vi "User Interface.vi"(10 "Test File Path":path=path "") -> ()   [LabVIEW 2020, in "Execution UI.lvclass"]
uses:
  Execution UI.lvclass
  Execution UI.lvclass/Execution UI.ctl
  <vilib>/Utility/miscctls.llb/LVNodeAndColumnTypeDef.ctl
  Private/TypeDefs/Execution State.ctl
  <vilib>/Platform/browser.llb/Open URL in Default Browser (string).vi
  Core/Result/Status.ctl
  Core/Result/Result.lvlib
  Result Model/Result Model.lvclass
  Core/Result/Type.ctl
  Core/Result/Result.ctl
  Framework/Test Finder/Test Finder.lvclass
  Framework/Test Runner/Test Runner.lvclass
  Configuration Manager/UI Configuration Manager.lvclass
  Result Model/Tree Item Filter.ctl
  Private/TypeDefs/Virtual Key.ctl
  Framework/Plugin/Plugin.lvclass
panel:
  in  "Refresh":bool
  in  "Run Selected Tests":bool
  in  "Stop":bool
  in  "Run All Tests":bool
  in  "Eject":bool
  in  "Collapse":bool
  in  "Expand":bool
  out "Progress bar":dbl(slide) scale=0.0..100.0
  out "Results":i32(listbox)=-1
  in  "Test Results":string[](tree)
  out "Shift?":bool
  in  "Filter fails":bool
  out "Description":string
  out "Status":string
  # "1"
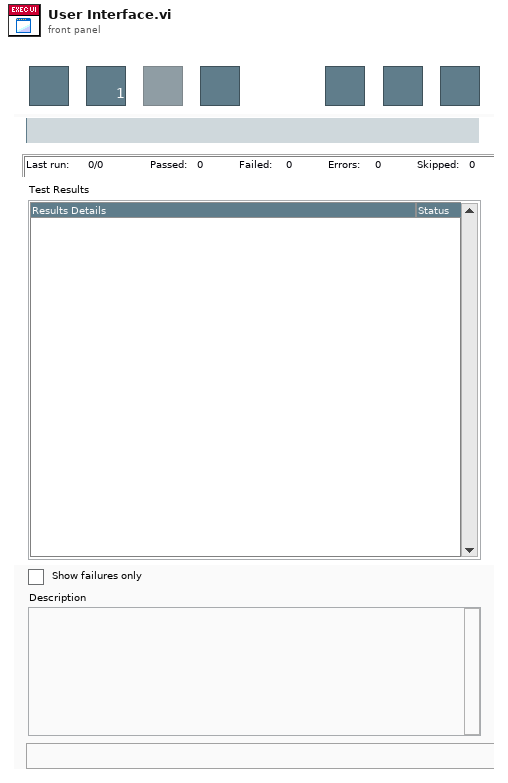
[diagram p1: front panel]
types:
  T1 = typedef "LVNodeAndColumnTypeDef.ctl" = cluster{"Node":string, "Column":i32}
  T2 = typedef "Result Model.lvclass/Tree Item Filter.ctl" = enum16{"All", "Only Fails", "Fails or else Not Executed"}
  T3 = cluster{"Text.Selection":cluster{"Selection Start":u32, "Selection End":u32}, "Color":u32}
  T4 = enum32{"Invalid", "Standard", "Closed", "Hidden", "Minimized", "Maximized"}
  T5 = typedef "Execution UI.lvclass/Execution State.ctl" = enum16{"Idle", "Running"}
  T6 = typedef "Result.lvlib/Result.ctl" = cluster{"Name":string, "Description":string, "Status":T7, "Result Type":T8, "Execution Time":dbl, "Data":cluster{"Expected":variant, "Actual":variant, "Delta":variant}}
  T7 = typedef "Result.lvlib/Status.ctl" = enum16{"", "Passed", "Failed", "Error", "Skipped", "Setup Error", "Broken", "Teardown Error"}
  T8 = typedef "Result.lvlib/Type.ctl" = enum16{"Test Case", "Test Suite", "Test Run", "Pass", "Fail", "Skip", "Pass if", "Fail if", "Pass if Error", "Fail if Error", "Pass if Equal", "Fail if Equal"}
  T9 = enum8{"Enabled", "Disabled", "Disabled and Grayed Out"}
  T10 = typedef "Execution UI.lvclass/Virtual Key.ctl" = enum16{"<None>", "Shift", "Ctrl", "Alt"}
  T11 = cluster{"Selection Start":u32, "Selection End":u32, "Type":enum16{"added", "missing"}}[]
  T12 = cluster{"Selection Start":u32, "Selection End":u32}
  T13 = typedef "Result Model.lvclass/Statistics.ctl" = cluster{"Method Count":u32, "Executed Methods":u32, "Passed Methods":u32, "Failed Methods":u32, "Method Errors":u32, "Skipped Method":u32, "Progress [%]":dbl}
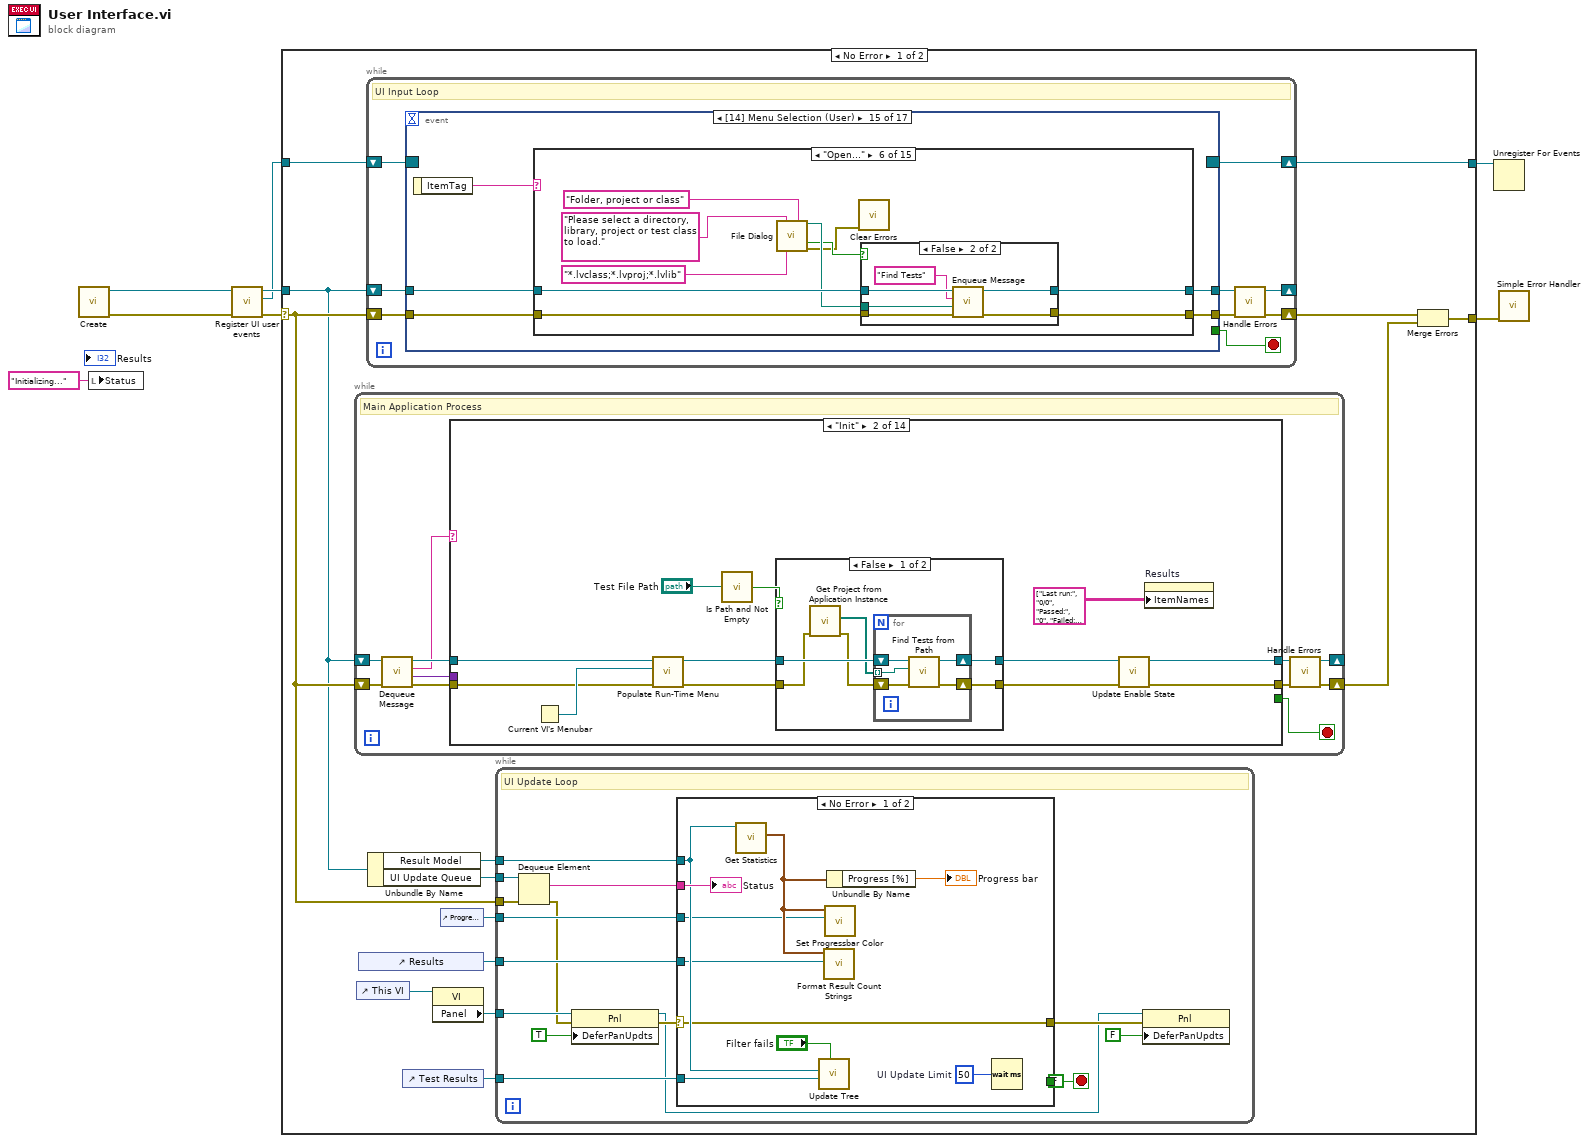
[diagram p0: block diagram]
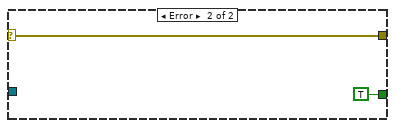
[diagram p2: hidden frame]
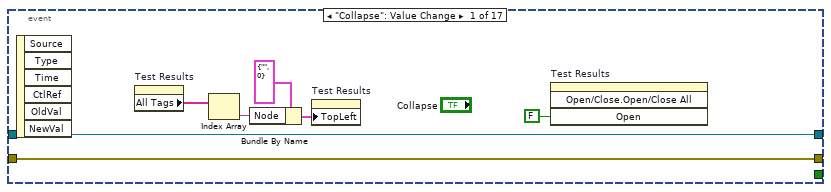
[diagram p3: hidden frame]
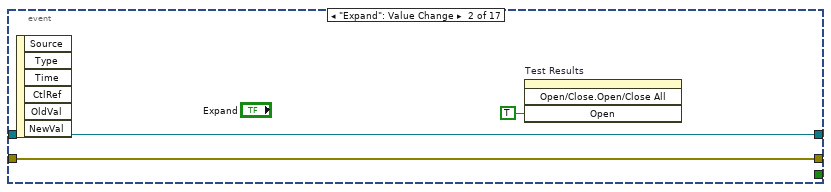
[diagram p4: hidden frame]
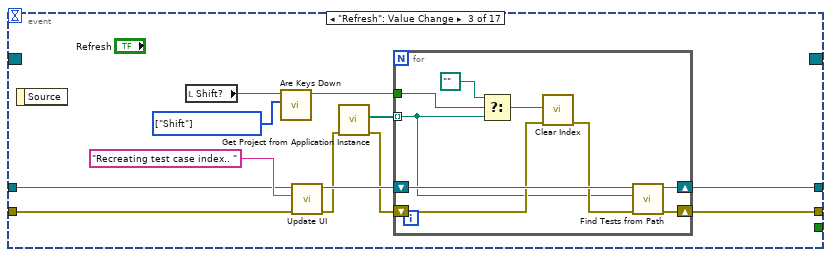
[diagram p5: hidden frame]
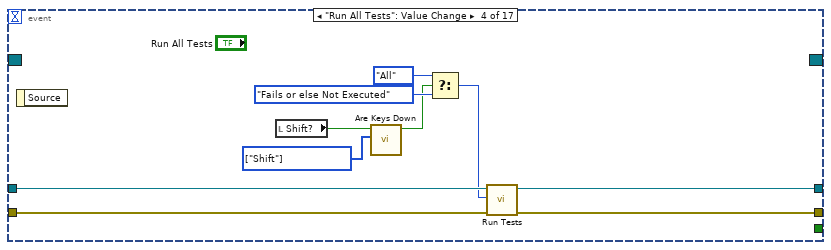
[diagram p6: hidden frame]
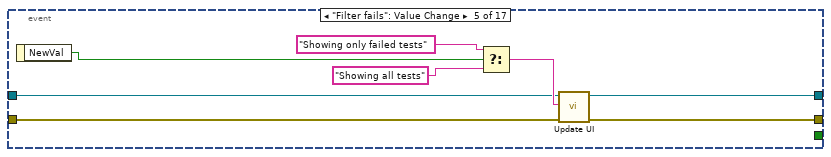
[diagram p7: hidden frame]
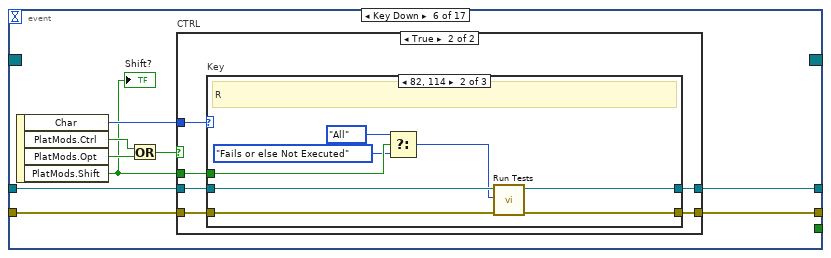
[diagram p8: hidden frame]
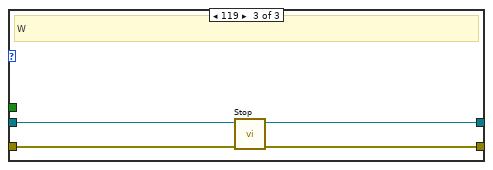
[diagram p11: hidden frame]
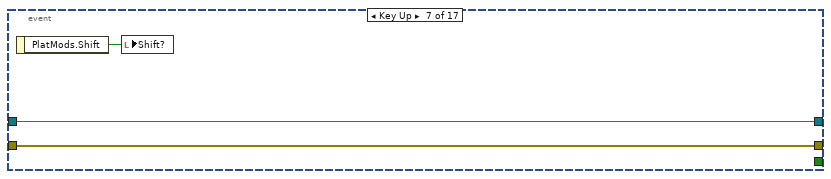
[diagram p12: hidden frame]
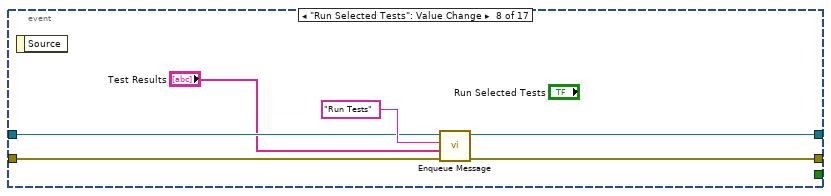
[diagram p13: hidden frame]
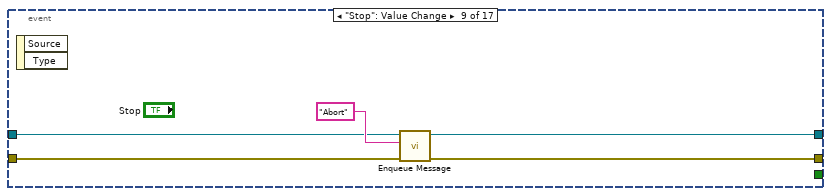
[diagram p14: hidden frame]
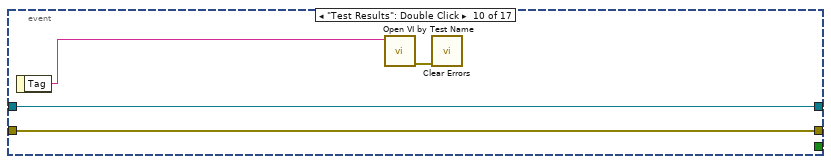
[diagram p15: hidden frame]
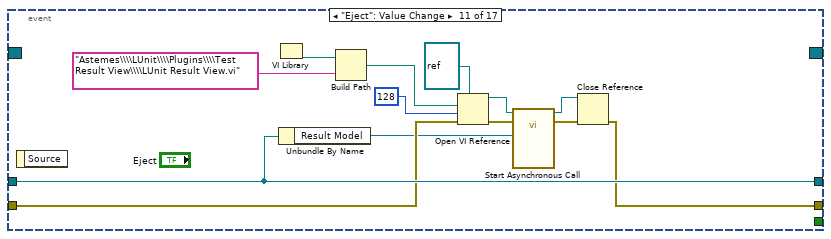
[diagram p16: hidden frame]
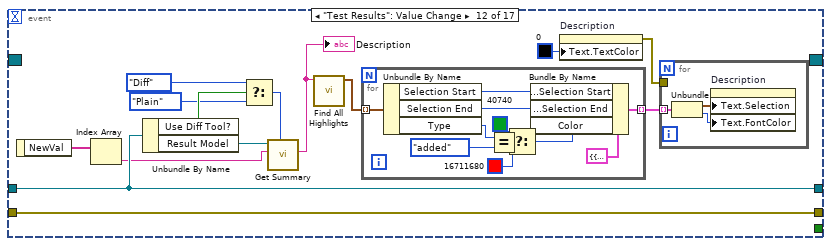
[diagram p17: hidden frame]
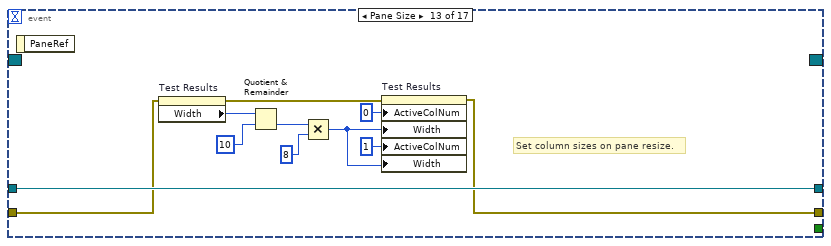
[diagram p18: hidden frame]
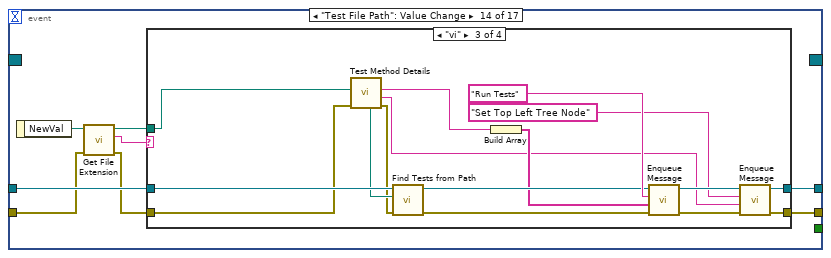
[diagram p19: hidden frame]
diagram:
  n1 = call "Create.vi"() -> ("error out"=w5:errorcluster, "Execution UI Out"=w6:refnum<class "Execution UI.lvclass">)  [unwired: 10 in]
  n2 = local write "Status"("Initializing..." ("Status")) -> ()
  n3 = call "Register UI user events.vi"("error in (no error)"=w5, "Execution UI In"=w6) -> ("error out"=w4:errorcluster, "Event Registration Refnum"=w7:refnum<event-registration>, "Execution UI Out"=w8:refnum<class "Execution UI.lvclass">)  [unwired: 7 in]
  n4 = case shown="No Error" w4 {
    selector: w4 -> [w14 w601]
    tunnel: w8 -> [w9 _]
    tunnel: w7 -> [w22 w602]
    tunnel: [w12 w601] -> w3
    tunnel: [w10 w602] -> w2
    frame No Error {
      n5 = while {
        shift-right: [w380] -> w13
        shift-left: w14 -> [w388]
        shift-right: [w382] -> _
        shift-left: w9 -> [w389]
        stop <- w385 stop-if-true
        # "Main Application Process"
        n6 = call "Dequeue Message.vi"("error in (no error)"=w388, "Process In"=w389) -> ("error out"=w386:errorcluster, "Message Data"=w383:variant, "Message"=w384:string, "Process Out"=w387:refnum<class "Execution UI.lvclass">)  [unwired: 6 in]
        n7 = case shown="\"Init\"" w384 {
          selector: w384 -> [w394 _ _ _ _ _ _ _ _ w535 w542 _ w578 _]
          tunnel: w387 -> [w395 w403 w436 w443 w454 w465 w485 w511 w519 w540 w544 w557 w582 w593]
          tunnel: [w395 w407 w423 w448 w455 w463 w486 w511 w519 w534 w547 w564 w589 refnum<class "Execution UI.lvclass"> refnum ("Execution UI Out")] -> w382
          tunnel: w386 -> [w396 w401 w430 w444 w459 w468 w494 w512 w520 w539 w551 w563 w588 w595]
          tunnel: [w397 w406 w425 w447 w458 w461 w488 w508 w520 w532 w545 w565 w590 w600] -> w381
          tunnel: [_ _ _ _ _ _ _ _ _ _ _ _ _ TRUE] -> w385
          tunnel: w383 -> [_ _ w433 w441 _ w466 w480 w510 _ w538 w550 w562 w587 _]
          frame Default {
            n8 = call <vilib>:"Get LV Class Name.vi"("object"=w395) -> ("class name"=w393:string)  [unwired: 9 in, 1 out]
            n9 = Format Into String(format string="Unknown command received in \"%s\": \"%s\"", w393, w394) -> (resulting string=w390:string)  [unwired: 2 in, 1 out]
            n10 = call <vilib>:"Error Cluster From Error Code.vi"("error in (no error)"=w396, "error message (\"\")"=w390, "error code (0)"=5004) -> ("error out"=w397:errorcluster)  [unwired: 6 in]
          }
          frame "Init" {
            n11 = Current VI's Menubar() -> (w404:refnum<k9>)
            n12 = call "Populate Run-Time Menu.vi"("error in (no error)"=w401, "Menu in"=w404, "Execution UI In"=w403) -> ("error out"=w402:errorcluster, "Execution UI Out"=w400:refnum<class "Execution UI.lvclass">)  [unwired: 7 in]
            n13 = call <vilib>:"Is Path and Not Empty.vi"("path"="Test File Path") -> ("Is Path and Not Empty?"=w398:bool)  [unwired: 4 in]
            n14 = case shown="False" w398 {
              tunnel: [w415 w422] -> w409
              tunnel: [w414 w421] -> w408
              tunnel: w402 -> [w411 w421]
              tunnel: w400 -> [w413 w422]
              frame False {
                n15 = call "Get Project from Application Instance.vi"("error in (no error)"=w411) -> ("error out"=w412:errorcluster, "Open Projects"=w410:path[])  [unwired: 9 in]
                n16 = for {
                  shift-right: [w420] -> w415
                  shift-left: w413 -> [w418]
                  shift-right: [w419] -> w414
                  shift-left: w412 -> [w417]
                  tunnel: w410 -> [w416] mode=indexing
                  n17 = call "Find Tests from Path.vi"("error in (no error)"=w417, "Test File Path"=w416, "Execution UI in"=w418) -> ("error out"=w419:errorcluster, "Execution UI out"=w420:refnum<class "Execution UI.lvclass">)  [unwired: 7 in]
                }
              }
              frame True {
              }
            }
            n18 = call "Update Enable State.vi"("error in (no error)"=w408, "Execution UI In"=w409) -> ("error out"=w406:errorcluster, "Execution UI Out"=w407:refnum<class "Execution UI.lvclass">)  [unwired: 8 in]
            n19 = property on="Results" class="MCListbox (strict)"("ItemNames"=string[][] [["Last run:", "0/0", "Passed:", "0", "Failed:", "0", "Errors:", "0", "Skipped:", "0"]] ("Result Texts")) -> ()  [unwired: 2 in, 2 out]
          }
          frame "Find Tests" {
            # "Error when calling from launcher because FP not opened."
            n20 = Variant To Data(error in=w430, type=path "" ("Not A Path Constant"), Variant=w433) -> (data=w431:path, error out=w429:errorcluster)
            n21 = call <vilib>:"Set Busy.vi"("error in (no error)"=w429) -> ("error out"=w435:errorcluster)  [unwired: 9 in, 1 out]
            n22 = call <vilib>:"Clear Errors.vi"("error in (no error)"=w435, "specific error code to clear (0: all)"=26) -> ("error out"=w428:errorcluster)  [unwired: 4 in, 1 out]
            n23 = call "Find Tests.vi"("error in (no error)"=w428, "Project or Class Path"=w431, "Execution UI In"=w436) -> ("error out"=w424:errorcluster, "Execution UI Out"=w423:refnum<class "Execution UI.lvclass">)  [unwired: 7 in]
            n24 = call <vilib>:"Unset Busy.vi"("error in (no error)"=w424) -> ("error out"=w434:errorcluster)  [unwired: 10 in]
            n25 = call <vilib>:"Clear Errors.vi"("error in (no error)"=w434, "specific error code to clear (0: all)"=26) -> ("error out"=w425:errorcluster)  [unwired: 4 in, 1 out]
          }
          frame "Run Tests" {
            # "[Test Case Class.lvclass:Test Method.vi] or [Test Case Class.lvclass]"
            n26 = Variant To Data(error in=w444, Variant=w441) -> (data=w440:string[], error out=w442:errorcluster)  [unwired: 1 in]
            n27 = call "Execute Tests.vi"("error in (no error)"=w442, "Tests"=w440, "Execution UI In"=w443) -> ("error out"=w445:errorcluster, "Execution UI Out"=w438:refnum<class "Execution UI.lvclass">)  [unwired: 7 in]
            n28 = call "Update Enable State.vi"("error in (no error)"=w445, "Execution UI In"=w438) -> ("error out"=w439:errorcluster, "Execution UI Out"=w437:refnum<class "Execution UI.lvclass">)  [unwired: 8 in]
            n29 = call "Update UI.vi"("error in (no error)"=w439, "Status"="Running tests...", "Execution UI In"=w437) -> ("error out"=w447:errorcluster, "Execution UI Out"=w448:refnum<class "Execution UI.lvclass">)  [unwired: 7 in]
          }
          frame "Abort" {
            n30 = Unbundle By Name(w454) -> ("Test Runner"=w452:refnum<class "Test Runner.lvclass">)
            n31 = call-dynamic "Abort.vi"("error in (no error)"=w459, "Test Runner in"=w452) -> ("error out"=w453:errorcluster)  [unwired: 9 in]
            n32 = Bundle By Name(cluster=w454, "Execution State"=Execution_State."Idle") -> (w450:refnum<class "Execution UI.lvclass">)
            n33 = call "Update Enable State.vi"("error in (no error)"=w453, "Execution UI In"=w450) -> ("error out"=w451:errorcluster, "Execution UI Out"=w449:refnum<class "Execution UI.lvclass">)  [unwired: 8 in]
            n34 = call "Update UI.vi"("error in (no error)"=w451, "Status"="Aborting tests", "Execution UI In"=w449) -> ("error out"=w458:errorcluster, "Execution UI Out"=w455:refnum<class "Execution UI.lvclass">)  [unwired: 7 in]
          }
          frame "Result" {
            n35 = Variant To Data(error in=w468, type=T6 {"Name"="", "Description"="", "Status"=enum."Passed", "Result Type"=enum."Test Suite", "Execution Time"=0.0, "Data"={"Expected"=variant, "Actual"=variant, "Delta"=variant}} ("Result"), Variant=w466) -> (data=w460:T6, error out=w462:errorcluster)
            n36 = in-place {
              in-place-border: w460 -> [w472]
              n37 = in-place-cluster #1(w465) -> ("Result Model"=w471:refnum<class "Result Model.lvclass">, "Plugins"=w470:refnum<class "Plugin.lvclass">[])
              n38 = call-dynamic "Result.vi"("Results"=w472, "Result Model by Reference In"=w471) -> ()  [unwired: 9 in, 1 out]
              n39 = for {
                tunnel: w472 -> [w475]
                tunnel: w470 -> [w474] mode=indexing
                tunnel: [w473] -> w469 mode=indexing
                n40 = call-dynamic "Result.vi"("Result"=w475, "Plugin In"=w474) -> ("Plugin Out"=w473:refnum<class "Plugin.lvclass">)  [unwired: 8 in, 1 out]
              }
              n41 = in-place-cluster #1("Result Model"=w471, "Plugins"=w469) -> (w464:refnum<class "Execution UI.lvclass">)
            }
            n42 = call "Update Status on Result.vi"("error in (no error)"=w462, "Result"=w460, "Execution UI V2 in"=w464) -> ("error out"=w461:errorcluster, "Execution UI V2 out"=w463:refnum<class "Execution UI.lvclass">)  [unwired: 7 in]
          }
          frame "Test Run Result" {
            n43 = Variant To Data(error in=w494, type=T6 {"Name"="", "Description"="", "Status"=enum."Passed", "Result Type"=enum."Test Suite", "Execution Time"=0.0, "Data"={"Expected"=variant, "Actual"=variant, "Delta"=variant}} ("Result"), Variant=w480) -> (data=w478:T6, error out=w481:errorcluster)
            n44 = Bundle By Name(cluster=w485, "Execution State"=Execution_State."Idle") -> (w477:refnum<class "Execution UI.lvclass">)
            n45 = local read "Test Results"() -> (w489:string[])
            n46 = in-place {
              in-place-border: w478 -> [w496]
              n47 = in-place-cluster #2(w477) -> ("Plugins"=w498:refnum<class "Plugin.lvclass">[], "Result Model"=w495:refnum<class "Result Model.lvclass">)
              n48 = call-dynamic "Result.vi"("Results"=w496, "Result Model by Reference In"=w495) -> ()  [unwired: 9 in, 1 out]
              n49 = for {
                tunnel: w496 -> [w503]
                tunnel: w498 -> [w501] mode=indexing
                tunnel: [w499] -> w497 mode=indexing
                n50 = call-dynamic "Result.vi"("Result"=w503, "Plugin In"=w501) -> ("error out"=w502:errorcluster, "Plugin Out"=w500:refnum<class "Plugin.lvclass">)  [unwired: 8 in]
                n51 = call-dynamic "Stop Test.vi"("error in (no error)"=w502, "Plugin in"=w500) -> ("Plugin out"=w499:refnum<class "Plugin.lvclass">)  [unwired: 8 in, 1 out]
              }
              n52 = in-place-cluster #2("Plugins"=w497, "Result Model"=w495) -> (w476:refnum<class "Execution UI.lvclass">)
            }
            n53 = property on="Test Results" class="Tree (strict)"("Val(Sgnl)"=w489) -> ()  [unwired: 2 in, 2 out]
            n54 = Unbundle By Name(w485) -> ("Start Time"=w483:timestamp)
            n55 = Get Date/Time In Seconds() -> (seconds since 1Jan1904=w484:timestamp)
            n56 = Subtract(x=w484, y=w483) -> (x-y=w482:dbl)
            n57 = Format Into String(format string="Finished in %.2f seconds", w482) -> (resulting string=w491:string)  [unwired: 2 in, 1 out]
            n58 = call "Update UI.vi"("error in (no error)"=w481, "Status"=w491, "Execution UI In"=w476) -> ("error out"=w493:errorcluster, "Execution UI Out"=w487:refnum<class "Execution UI.lvclass">)  [unwired: 7 in]
            n59 = call "Update Enable State.vi"("error in (no error)"=w493, "Execution UI In"=w487) -> ("error out"=w488:errorcluster, "Execution UI Out"=w486:refnum<class "Execution UI.lvclass">)  [unwired: 8 in]
          }
          frame "Set Top Left Tree Node" {
            n60 = Variant To Data(error in=w512, type="", Variant=w510) -> (data=w504:string, error out=w508:errorcluster)
            n61 = control-ref of="Test Results"() -> (w507:refnum<vi>)
            n62 = Bundle By Name(cluster=T1 {"Node"="", "Column"=0} ("Top Left Visible Cell"), "Node"=w504) -> (w505:T1)
            n63 = property on="Property Node" class="Tree (strict)"(reference=w507, "TopLeft"=w505) -> ()  [unwired: 1 in, 2 out]
          }
          frame "Update Enable State" {
            n64 = Unbundle By Name(w519) -> ("Execution State"=w518:T5)
            n65 = case shown="\"Running\"" w518 {
              tunnel: [T9."Enabled" ("Disabled") T9."Disabled and Grayed Out" ("Disabled")] -> w517
              tunnel: [T9."Disabled and Grayed Out" ("Disabled") T9."Enabled" ("Disabled")] -> w516
              tunnel: [T9."Disabled and Grayed Out" ("Disabled") T9."Enabled" ("Disabled")] -> w515
              tunnel: [T9."Disabled and Grayed Out" ("Disabled") T9."Enabled" ("Disabled")] -> w514
              tunnel: [T9."Disabled and Grayed Out" ("Disabled") T9."Enabled" ("Disabled")] -> w513
              frame "Running" {
              }
              frame "Idle" {
              }
            }
            n66 = property on="Stop" class="Bool"("DisabledEnum"=w517) -> ()  [unwired: 2 in, 2 out]
            n67 = property on="Run Selected Tests" class="Bool"("DisabledEnum"=w516) -> ()  [unwired: 2 in, 2 out]
            n68 = property on="Run All Tests" class="Bool"("DisabledEnum"=w515) -> ()  [unwired: 2 in, 2 out]
            n69 = property on="Refresh" class="Bool"("DisabledEnum"=w514) -> ()  [unwired: 2 in, 2 out]
            n70 = property on="Eject" class="Bool"("DisabledEnum"=w513) -> ()  [unwired: 2 in, 2 out]
          }
          frame "Ignore Dashed Tests" {
            n71 = Variant To Data(error in=w539, type=FALSE, Variant=w538) -> (data=w531:bool, error out=w533:errorcluster)
            n72 = Current VI's Menubar() -> (w536:refnum<k9>)
            n73 = Set Menu Item Info(6:w531, 7:w535, 11:w536) -> ()  [unwired: 4 in, 2 out]
            n74 = Bundle By Name(cluster=w540, "Ignore Dashed Tests?"=w531) -> (w534:refnum<class "Execution UI.lvclass">)
            n75 = call "Set Dashed Tests Ignored.vi"("error in (no error)"=w533, "Ingore Dashed?"=w531) -> ("error out"=w532:errorcluster)  [unwired: 9 in]
          }
          frame "Run Tests in Parallel" {
            w543 = TRUE  # Persist?
            n76 = Variant To Data(error in=w551, type=FALSE, Variant=w550) -> (data=w541:bool, error out=w546:errorcluster)
            n77 = Current VI's Menubar() -> (w548:refnum<k9>)
            n78 = Set Menu Item Info(6:w541, 7:w542, 11:w548) -> ()  [unwired: 4 in, 2 out]
            n79 = call "Configure Parallel Execution.vi"("error in (no error)"=w546, "Persist?"=w543, "Enable Parallel Execution?"=w541, "Execution UI In"=w544) -> ("error out"=w545:errorcluster, "Execution UI Out"=w547:refnum<class "Execution UI.lvclass">)  [unwired: 6 in]
          }
          frame "Execution Profiler..." {
            n80 = Variant To Data(error in=w563, type=TRUE, Variant=w562) -> (data=w552:bool, error out=w556:errorcluster)
            n81 = Select(t="Run a test to generate an execution analysis." ("Status"), s=w552, f="Execution profiler disabled" ("Status")) -> (s? t:f=w558:string)
            n82 = case shown="False" w552 {
              tunnel: [w570 w572] -> w554
              tunnel: w557 -> [w569 w575]
              tunnel: w556 -> [w568 w574]
              tunnel: [w567 w573] -> w555
              tunnel: "Execution Profiler.lvclass" -> [w566 w571]
              frame False {
                n83 = call "Clear Plugin.vi"("error in (no error)"=w568, "Plugin"=w566, "Execution UI in"=w569) -> ("error out"=w567:errorcluster, "Execution UI out"=w570:refnum<class "Execution UI.lvclass">)  [unwired: 7 in]
              }
              frame True {
                n84 = call "Init Plugin.vi"("error in (no error)"=w574, "Plugin"=w571, "Execution UI in"=w575) -> ("error out"=w573:errorcluster, "Execution UI out"=w572:refnum<class "Execution UI.lvclass">)  [unwired: 7 in]
              }
            }
            n85 = call "Update UI.vi"("error in (no error)"=w555, "Status"=w558, "Execution UI In"=w554) -> ("error out"=w565:errorcluster, "Execution UI Out"=w564:refnum<class "Execution UI.lvclass">)  [unwired: 7 in]
          }
          frame "Reporting..." {
            n86 = Variant To Data(error in=w588, type=TRUE, Variant=w587) -> (error out=w580:errorcluster)  [unwired: 1 out]
            n87 = call "Configure Reporting Dialog.vi"("error in (no error)"=w580, "Execution UI In"=w582) -> ("error out"=w579:errorcluster, "Reporting Enabled?"=w576:bool, "Execution UI Out"=w581:refnum<class "Execution UI.lvclass">)  [unwired: 7 in]
            n88 = Current VI's Menubar() -> (w577:refnum<k9>)
            n89 = Set Menu Item Info(6:w576, 7:w578, 11:w577) -> ()  [unwired: 4 in, 2 out]
            n90 = Select(t="Run a test to generate a report." ("Status"), s=w576, f="Report generation disabled" ("Status")) -> (s? t:f=w583:string)
            n91 = call "Update UI.vi"("error in (no error)"=w579, "Status"=w583, "Execution UI In"=w581) -> ("error out"=w590:errorcluster, "Execution UI Out"=w589:refnum<class "Execution UI.lvclass">)  [unwired: 7 in]
          }
          frame "Stop" {
            n92 = control-ref of="This VI"() -> (w598:refnum<vi>)
            n93 = invoke on="Invoke Node" class="VI" method="FP.Close"(reference=w598, error in=w595) -> (reference out=w596:refnum<vi>, error out=w597:errorcluster)  [unwired: 1 in, 1 out]
            n94 = Close Reference(reference=w596, error in (no error)=w597) -> (error out=w591:errorcluster)
            n95 = Unbundle By Name(w593) -> ("Test Runner"=w592:refnum<class "Test Runner.lvclass">)
            n96 = call-dynamic "Abort.vi"("Test Runner in"=w592) -> ()  [unwired: 10 in, 1 out]
            n97 = call-dynamic "Clear.vi"("error in (no error)"=w591, "Execution UI In"=w593) -> ("error out"=w600:errorcluster)  [unwired: 9 in]
          }
        }
        n98 = call "Handle Errors.vi"("error in (no error)"=w381) -> ("error out"=w380:errorcluster)  [unwired: 10 in]
      }
      n99 = control-ref of="This VI"() -> (w19:refnum<vi>)
      n100 = control-ref of="Results"() -> (w16:refnum<vi>)
      n101 = while {
        shift-right: [w51] -> w11
        shift-left: w14 -> [w57]
        shift-right: [w53] -> _
        shift-left: w9 -> [w58]
        shift-right: [w55] -> w10
        shift-left: w22 -> [w54]
        stop <- w56 stop-if-true
        # "UI Input Loop"
        n102 = event shown="[14] Menu Selection (User)" {
          selector: w54 -> [_ _ _ _ _ _ _ _ _ _ _ _ _ _ _ _ _]
          dyn-events: [_ _ _ _ _ _ _ _ _ _ _ _ _ _ _ _ _] -> w55
          timeout: _ -> [_ _ _ _ _ _ _ _ _ _ _ _ _ _ _ _ _]
          tunnel: w58 -> [w64 w67 w79 w97 w101 w115 w140 w144 w149 w156 w164 w182 w208 w216 w263 w372 w378]
          tunnel: w57 -> [w65 w68 w78 w96 w103 w116 w141 w146 w152 w155 w159 w183 w198 w209 w262 w373 w375]
          tunnel: [w65 w68 w77 w99 w104 w114 w141 w147 w151 w155 w163 w183 w199 w214 w261 w373 w376] -> w52
          tunnel: [w64 w67 w75 w98 w102 w113 w140 w143 w148 w156 w164 w182 w208 w213 w260 w372 w377] -> w53
          tunnel: [_ _ _ _ _ _ _ _ _ _ _ _ _ _ _ TRUE _] -> w56
          event "Collapse": Value Change {
            n103 = event-data() -> ()  [unwired: 1 in, 6 out]
            n104 = property on="Test Results" class="Tree (strict)"() -> ("All Tags"=w62:string[])  [unwired: 2 in, 2 out]
            n105 = Index Array(array=w62) -> (element=w59:string)  [unwired: 1 in]
            n106 = Bundle By Name(cluster=T1 {"Node"="", "Column"=0} ("Top Left Visible Cell"), "Node"=w59) -> (w60:T1)
            n107 = property on="Test Results" class="Tree (strict)"("TopLeft"=w60) -> ()  [unwired: 2 in, 2 out]
            n108 = invoke on="Test Results" class="Tree (strict)" method="Open/Close.Open/Close All"("Open"=FALSE ("Open?")) -> ()  [unwired: 3 in, 4 out]
          }
          event "Expand": Value Change {
            n109 = event-data() -> ()  [unwired: 1 in, 6 out]
            n110 = invoke on="Test Results" class="Tree (strict)" method="Open/Close.Open/Close All"("Open"=TRUE ("Open?")) -> ()  [unwired: 3 in, 4 out]
          }
          event "Refresh": Value Change {
            w71 = T10[] [enum."Shift"] items=["<None>", "Shift", "Ctrl", "Alt"] ("Virtual Keys")
            n111 = event-data() -> ()  [unwired: 1 in, 1 out]
            n112 = local read "Shift?"() -> (w70:bool)
            n113 = call "Are Keys Down.vi"("Keys"=w71, "Fallback Value (Mac only)"=w70) -> ("Are Keys Down?"=w69:bool)  [unwired: 8 in, 1 out]
            n114 = call "Update UI.vi"("error in (no error)"=w78, "Status"="Recreating test case index.. ", "Execution UI In"=w79) -> ("error out"=w74:errorcluster, "Execution UI Out"=w76:refnum<class "Execution UI.lvclass">)  [unwired: 7 in]
            n115 = call "Get Project from Application Instance.vi"("error in (no error)"=w74) -> ("error out"=w73:errorcluster, "Open Projects"=w72:path[])  [unwired: 9 in]
            n116 = for {
              tunnel: w72 -> [w82] mode=indexing
              shift-right: [w87] -> w75
              shift-left: w76 -> [w88]
              shift-right: [w89] -> w77
              shift-left: w73 -> [w85]
              tunnel: w69 -> [w83]
              n117 = Select(t=path "" ("Path"), s=w83, f=w82) -> (s? t:f=w81:path)
              n118 = call "Clear Index.vi"("error in (no error)"=w85, "Project Path"=w81) -> ("error out"=w86:errorcluster)  [unwired: 9 in]
              n119 = call "Find Tests from Path.vi"("error in (no error)"=w86, "Test File Path"=w82, "Execution UI in"=w88) -> ("error out"=w89:errorcluster, "Execution UI out"=w87:refnum<class "Execution UI.lvclass">)  [unwired: 7 in]
            }
          }
          event "Run All Tests": Value Change {
            w90 = T10[] [enum."Shift"] items=["<None>", "Shift", "Ctrl", "Alt"] ("Virtual Keys")
            n120 = event-data() -> ()  [unwired: 1 in, 1 out]
            n121 = local read "Shift?"() -> (w92:bool)
            n122 = call "Are Keys Down.vi"("Keys"=w90, "Fallback Value (Mac only)"=w92) -> ("Are Keys Down?"=w91:bool)  [unwired: 8 in, 1 out]
            n123 = Select(t=Tree_Item_Filter."All" ("Filter"), s=w91, f=Tree_Item_Filter."Fails or else Not Executed") -> (s? t:f=w94:T2)
            n124 = call "Run Tests.vi"("error in (no error)"=w96, "Filter"=w94, "Execution UI in"=w97) -> ("error out"=w99:errorcluster, "Execution UI out"=w98:refnum<class "Execution UI.lvclass">)  [unwired: 7 in]
          }
          event "Filter fails": Value Change {
            n125 = event-data() -> ("NewVal"=w100:bool)  [unwired: 1 in]
            n126 = Select(t="Showing only failed tests", s=w100, f="Showing all tests") -> (s? t:f=w107:string)
            n127 = call "Update UI.vi"("error in (no error)"=w103, "Status"=w107, "Execution UI In"=w101) -> ("error out"=w104:errorcluster, "Execution UI Out"=w102:refnum<class "Execution UI.lvclass">)  [unwired: 7 in]
          }
          event Key Down {
            n128 = event-data() -> ("Char"=w109:i16, "PlatMods.Ctrl"=w112:bool, "PlatMods.Opt"=w111:bool, "PlatMods.Shift"=w108:bool)  [unwired: 1 in]
            "Shift?" <- w108
            n129 = Or(x=w112, y=w111) -> (x .or. y?=w110:bool)
            n130 = case "CTRL" shown="True" w110 {
              tunnel: w116 -> [w117 w124]
              tunnel: w115 -> [w118 w123]
              tunnel: [w117 w122] -> w114
              tunnel: [w118 w121] -> w113
              tunnel: w109 -> [_ w120]
              tunnel: w108 -> [_ w119]
              frame False {
              }
              frame True {
                n131 = case "Key" shown="82, 114" w120 {
                  tunnel: w124 -> [w125 w133 w137]
                  tunnel: w123 -> [w126 w134 w138]
                  tunnel: [w125 w131 w135] -> w122
                  tunnel: [w126 w132 w136] -> w121
                  tunnel: w119 -> [_ w130 _]
                  frame Default {
                  }
                  frame 82, 114 {
                    # "R"
                    n132 = Select(t=Tree_Item_Filter."All" ("Filter"), s=w130, f=Tree_Item_Filter."Fails or else Not Executed" ("Filter")) -> (s? t:f=w127:T2)
                    n133 = call "Run Tests.vi"("error in (no error)"=w133, "Filter"=w127, "Execution UI in"=w134) -> ("error out"=w131:errorcluster, "Execution UI out"=w132:refnum<class "Execution UI.lvclass">)  [unwired: 7 in]
                  }
                  frame 119 {
                    # "W"
                    n134 = call-dynamic "Stop.vi"("error in (no error)"=w137, "Execution UI In"=w138) -> ("error out"=w135:errorcluster, "Execution UI Out"=w136:refnum<class "Execution UI.lvclass">)  [unwired: 8 in]
                  }
                }
              }
            }
          }
          event Key Up {
            n135 = event-data() -> ("PlatMods.Shift"=w139:bool)  [unwired: 1 in]
            n136 = local write "Shift?"(w139) -> ()
          }
          event "Run Selected Tests": Value Change {
            n137 = event-data() -> ()  [unwired: 1 in, 1 out]
            n138 = call "Enqueue Message.vi"("error in (no error)"=w146, "Message Data"="Test Results", "Message"="Run Tests", "Process In"=w144) -> ("error out"=w147:errorcluster, "Process Out"=w143:refnum<class "Execution UI.lvclass">)  [unwired: 6 in]
          }
          event "Stop": Value Change {
            n139 = event-data() -> ()  [unwired: 1 in, 2 out]
            n140 = call "Enqueue Message.vi"("error in (no error)"=w152, "Message"="Abort", "Process In"=w149) -> ("error out"=w151:errorcluster, "Process Out"=w148:refnum<class "Execution UI.lvclass">)  [unwired: 7 in]
          }
          event "Test Results": Double Click {
            n141 = event-data() -> ("Tag"=w154:string)  [unwired: 1 in]
            n142 = call "Open VI by Test Name.vi"("Tag"=w154) -> ("error in (no error) 2"=w153:errorcluster)  [unwired: 10 in]
            n143 = call <vilib>:"Clear Errors.vi"("error in (no error)"=w153) -> ()  [unwired: 5 in, 2 out]
          }
          event "Eject": Value Change {
            n144 = event-data() -> ()  [unwired: 1 in, 1 out]
            n145 = VI Library() -> (path=w161:path)
            n146 = Unbundle By Name(w164) -> ("Result Model"=w157:refnum<class "Result Model.lvclass">)
            n147 = Build Path(base path=w161, name or relative path="Astemes\\\\LUnit\\\\Plugins\\\\Test Result View\\\\LUnit Result View.vi" ("Relative Path from 1 to 2")) -> (appended path=w160:path)
            n148 = Open VI Reference(type specifier VI Refnum (for type only)=refnum<vi> refnum, vi path=w160, options=128, error in (no error)=w159) -> (vi reference=w169:refnum<vi>, error out=w168:errorcluster)  [unwired: 2 in]
            n149 = call-by-ref "Start Asynchronous Call"(reference=w169, error in=w168, "Result Model"=w157) -> (reference out=w167:refnum<vi>, error out=w166:errorcluster)  [unwired: 11 in]
            n150 = Close Reference(reference=w167, error in (no error)=w166) -> (error out=w163:errorcluster)
          }
          event "Test Results": Value Change {
            n151 = event-data() -> ("NewVal"=w181:string[])  [unwired: 1 in]
            n152 = Index Array(array=w181) -> (element=w180:string)  [unwired: 1 in]
            n153 = Unbundle By Name(w182) -> ("Use Diff Tool?"=w173:bool, "Result Model"=w179:refnum<class "Result Model.lvclass">)
            n154 = Select(t=enum16{"Diff", "Plain"}."Diff" ("Style"), s=w173, f=enum16{"Diff", "Plain"}."Plain" ("Style")) -> (s? t:f=w171:enum16{"Diff", "Plain"})
            n155 = call "Get Summary.vi"("Style"=w171, "Item"=w180, "Result Model by Reference In"=w179) -> ("Summary"=w175:string)  [unwired: 7 in, 1 out]
            "Description" <- w175
            n156 = call "Find All Highlights.vi"("String"=w175) -> ("Sections"=w174:T11)  [unwired: 10 in]
            n157 = for {
              tunnel: w174 -> [w194] mode=indexing
              tunnel: [w188] -> w178 mode=indexing
              n158 = Unbundle By Name(w194) -> ("Selection Start"=w192:u32, "Selection End"=w191:u32, "Type"=w190:enum16{"added", "missing"})
              n159 = Equal?(x=w190, y=enum16{"added", "missing"}."added") -> (x = y?=w187:bool)
              n160 = Select(t=u32 40740 ("Text.Text Colors:Text Color"), s=w187, f=u32 16711680 ("Text.Text Colors:Text Color")) -> (s? t:f=w184:u32)
              n161 = Bundle By Name(cluster=T3 {"Text.Selection"={"Selection Start"=0, "Selection End"=0}, "Color"=40740} ("Colors"), "Text.Selection.Selection Start"=w192, "Text.Selection.Selection End"=w191, "Color"=w184) -> (w188:T3)
            }
            n162 = property on="Description" class="Str"("Text.TextColor"=u32 0 ("Text.Text Colors:Text Color")) -> (error out=w177:errorcluster)  [unwired: 2 in, 1 out]
            n163 = for {
              tunnel: w178 -> [w195] mode=indexing
              tunnel: w177 -> [_]
              n164 = Unbundle(w195) -> ("Text.Selection"=w197:T12, "Color"=w196:u32)
              n165 = property on="Description" class="Str"("Text.Selection"=w197, "Text.FontColor"=w196) -> ()  [unwired: 2 in, 2 out]
            }
          }
          event Pane Size {
            # "Set column sizes on pane resize."
            n166 = event-data() -> ()  [unwired: 1 in, 1 out]
            n167 = property on="Test Results" class="Tree (strict)"(error in=w198) -> (error out=w200:errorcluster, "Width"=w201:u32)  [unwired: 1 in, 1 out]
            n168 = Quotient & Remainder(x=w201, y=u32 10) -> (floor(x/y)=w205:u32)  [unwired: 1 out]
            n169 = Multiply(x=w205, y=u32 8) -> (x*y=w202:u32)
            n170 = property on="Test Results" class="Tree (strict)"(error in=w200, "ActiveColNum"=0 ("Active Cell:Active Column Number"), "Width"=w202, "ActiveColNum"=1 ("Active Cell:Active Column Number"), "Width"=w202) -> (error out=w199:errorcluster)  [unwired: 1 in, 1 out]
          }
          event "Test File Path": Value Change {
            n171 = event-data() -> ("NewVal"=w215:path)  [unwired: 1 in]
            n172 = call <vilib>:"Get File Extension.vi"("error in (no error)"=w209, "file"=w215) -> ("error out"=w210:errorcluster, "lowercase file extension"=w211:string, "dup file"=w212:path)  [unwired: 5 in, 2 out]
            n173 = case shown="\"vi\"" w211 {
              tunnel: w216 -> [w218 w234 w250 w259]
              tunnel: w210 -> [w217 w233 w238 w258]
              tunnel: w212 -> [_ w229 w240 w257]
              tunnel: [w217 w224 w245 w254] -> w214
              tunnel: [w218 w222 w243 w253] -> w213
              frame Default {
              }
              frame "lvclass" {
                n174 = call "Find Tests from Path.vi"("error in (no error)"=w233, "Test File Path"=w229, "Execution UI in"=w234) -> ("error out"=w227:errorcluster, "Execution UI out"=w228:refnum<class "Execution UI.lvclass">)  [unwired: 7 in]
                n175 = call <vilib>:"Get LV Class Default Value.vi"("error in (no error)"=w227, "class path"=w229) -> ("error out"=w231:errorcluster, "object"=w230:refnum<class>)  [unwired: 8 in]
                n176 = call <vilib>:"Get LV Class Name.vi"("error in (no error)"=w231, "object"=w230) -> ("error out"=w226:errorcluster, "class name"=w221:string)  [unwired: 8 in]
                n177 = Build Array(w221) -> (w219:string[])
                n178 = call "Enqueue Message.vi"("error in (no error)"=w226, "Message Data"=w219, "Message"="Run Tests", "Process In"=w228) -> ("error out"=w225:errorcluster, "Process Out"=w223:refnum<class "Execution UI.lvclass">)  [unwired: 6 in]
                n179 = call "Enqueue Message.vi"("error in (no error)"=w225, "Message Data"=w221, "Message"="Set Top Left Tree Node", "Process In"=w223) -> ("error out"=w224:errorcluster, "Process Out"=w222:refnum<class "Execution UI.lvclass">)  [unwired: 6 in]
              }
              frame "vi" {
                n180 = call "Test Method Details.vi"("error in (no error)"=w238, "vi path"=w240) -> ("error out"=w237:errorcluster, "Test Case Class"=w235:string, "Test Method"=w236:string, "Test Case Path"=w239:path)  [unwired: 6 in]
                n181 = call "Find Tests from Path.vi"("error in (no error)"=w237, "Test File Path"=w239, "Execution UI in"=w250) -> ("error out"=w247:errorcluster, "Execution UI out"=w248:refnum<class "Execution UI.lvclass">)  [unwired: 7 in]
                n182 = Build Array(w236) -> (w241:string[])
                n183 = call "Enqueue Message.vi"("error in (no error)"=w247, "Message Data"=w241, "Message"="Run Tests", "Process In"=w248) -> ("error out"=w246:errorcluster, "Process Out"=w244:refnum<class "Execution UI.lvclass">)  [unwired: 6 in]
                n184 = call "Enqueue Message.vi"("error in (no error)"=w246, "Message Data"=w235, "Message"="Set Top Left Tree Node", "Process In"=w244) -> ("error out"=w245:errorcluster, "Process Out"=w243:refnum<class "Execution UI.lvclass">)  [unwired: 6 in]
              }
              frame "lvproj" {
                n185 = call "Find Tests from Path.vi"("error in (no error)"=w258, "Test File Path"=w257, "Execution UI in"=w259) -> ("error out"=w255:errorcluster, "Execution UI out"=w256:refnum<class "Execution UI.lvclass">)  [unwired: 7 in]
                n186 = call "Enqueue Message.vi"("error in (no error)"=w255, "Message Data"=string[] [] ("data"), "Message"="Run Tests", "Process In"=w256) -> ("error out"=w254:errorcluster, "Process Out"=w253:refnum<class "Execution UI.lvclass">)  [unwired: 6 in]
              }
            }
          }
          event Menu Selection (User) {
            n187 = event-data() -> ("ItemTag"=w264:string)  [unwired: 1 in]
            n188 = case shown="\"Open...\"" w264 {
              selector: w264 -> [_ _ _ _ w301 _ w330 w337 w343 _ _ _ _ _ _]
              tunnel: w263 -> [w278 w280 w287 w299 w307 w315 w332 w339 w345 w350 w357 w361 w365 w366 w371]
              tunnel: w262 -> [w265 w279 w284 w293 w305 w316 w331 w341 w347 w352 w354 w358 w362 w367 w370]
              tunnel: [w266 w279 w282 w298 w303 w317 w329 w340 w346 w351 w355 w359 w363 w367 w369] -> w261
              tunnel: [w278 w280 w283 w297 w304 w318 w328 w338 w344 w350 w357 w361 w365 w366 w368] -> w260
              frame "Full Size" {
                n189 = control-ref of="This VI"() -> (w277:refnum<vi>)
                n190 = property on="Property Node" class="VI"(reference=w277, error in=w265, "FP.State"=T4."Maximized" ("Front Panel Window:State")) -> (error out=w268:errorcluster)  [unwired: 1 out]
                n191 = property on="Test Results" class="Tree (strict)"(error in=w268) -> (error out=w267:errorcluster, "Width"=w275:u32)  [unwired: 1 in, 1 out]
                n192 = Quotient & Remainder(x=w275, y=u32 10) -> (floor(x/y)=w274:u32)  [unwired: 1 out]
                n193 = Multiply(x=w274, y=u32 7) -> (x*y=w273:u32)
                n194 = property on="Test Results" class="Tree (strict)"(error in=w267, "ActiveColNum"=0 ("Active Cell:Active Column Number"), "Width"=w273, "ActiveColNum"=1 ("Active Cell:Active Column Number"), "Width"=w273) -> (error out=w266:errorcluster)  [unwired: 1 in, 1 out]
              }
              frame Default {
              }
              frame "Ignore Dashed Tests" {
                w286 = "Ignore Dashed Tests"
                n195 = Current VI's Menubar() -> (w288:refnum<k9>)
                n196 = Get Menu Item Info(7:w286, 11:w288) -> (4:w285:bool)  [unwired: 1 in, 6 out]
                n197 = Not(x=w285) -> (.not. x?=w281:bool)
                n198 = call "Enqueue Message.vi"("error in (no error)"=w284, "Message Data"=w281, "Message"=w286, "Process In"=w287) -> ("error out"=w282:errorcluster, "Process Out"=w283:refnum<class "Execution UI.lvclass">)  [unwired: 6 in]
              }
              frame "Use Diff Tool" {
                w295 = "Use Diff Tool"
                n199 = property on="Test Results" class="Tree (strict)"() -> ("Value"=w291:string[])  [unwired: 2 in, 2 out]
                n200 = property on="Test Results" class="Tree (strict)"("Val(Sgnl)"=w291) -> ()  [unwired: 2 in, 2 out]
                n201 = Current VI's Menubar() -> (w300:refnum<k9>)
                n202 = Get Menu Item Info(7:w295, 8:w293, 11:w300) -> (0:w292:errorcluster, 3:w296:refnum<k9>, 4:w294:bool)  [unwired: 4 out]
                n203 = Not(x=w294) -> (.not. x?=w290:bool)
                n204 = Set Menu Item Info(6:w290, 7:w295, 8:w292, 11:w296) -> (0:w289:errorcluster)  [unwired: 3 in, 1 out]
                n205 = Bundle By Name(cluster=w299, "Use Diff Tool?"=w290) -> (w297:refnum<class "Execution UI.lvclass">)
                n206 = call "Set Use Diff Tool.vi"("error in (no error)"=w289, "Use Diff Tool?"=w290) -> ("error out"=w298:errorcluster)  [unwired: 9 in]
              }
              frame "Run Tests in Parallel" {
                n207 = Current VI's Menubar() -> (w308:refnum<k9>)
                n208 = Get Menu Item Info(7:w301, 11:w308) -> (4:w306:bool)  [unwired: 1 in, 6 out]
                n209 = Not(x=w306) -> (.not. x?=w302:bool)
                n210 = call "Enqueue Message.vi"("error in (no error)"=w305, "Message Data"=w302, "Message"=w301, "Process In"=w307) -> ("error out"=w303:errorcluster, "Process Out"=w304:refnum<class "Execution UI.lvclass">)  [unwired: 6 in]
              }
              frame "Open..." {
                n211 = call "File Dialog"("prompt"="Please select a directory, library, project or test class to load.", "pattern (all files)"="*.lvclass;*.lvproj;*.lvlib", "pattern label"="Folder, project or class") -> ("selected path"=w314:path, "cancelled"=w310:bool, "error out"=w309:errorcluster)  [unwired: 9 in, 1 out]
                n212 = call <vilib>:"Clear Errors.vi"("error in (no error)"=w309) -> ()  [unwired: 5 in, 2 out]
                n213 = case shown="False" w310 {
                  tunnel: [w320 w326] -> w318
                  tunnel: [w319 w325] -> w317
                  tunnel: w316 -> [w319 w324]
                  tunnel: w315 -> [w320 w323]
                  tunnel: w314 -> [_ w322]
                  frame True {
                  }
                  frame False {
                    n214 = call "Enqueue Message.vi"("error in (no error)"=w324, "Message Data"=w322, "Message"="Find Tests", "Process In"=w323) -> ("error out"=w325:errorcluster, "Process Out"=w326:refnum<class "Execution UI.lvclass">)  [unwired: 6 in]
                  }
                }
              }
              frame "Reporting..." {
                n215 = Current VI's Menubar() -> (w327:refnum<k9>)
                n216 = Get Menu Item Info(7:w330, 8:w331, 11:w327) -> (0:w335:errorcluster, 4:w333:bool)  [unwired: 5 out]
                n217 = Not(x=w333) -> (.not. x?=w334:bool)
                n218 = call "Enqueue Message.vi"("error in (no error)"=w335, "Message Data"=w334, "Message"=w330, "Process In"=w332) -> ("error out"=w329:errorcluster, "Process Out"=w328:refnum<class "Execution UI.lvclass">)  [unwired: 6 in]
              }
              frame "Execution Profiler..." {
                n219 = Current VI's Menubar() -> (w336:refnum<k9>)
                n220 = call "Toggle Plugin.vi"("menu reference"=w336, "error in (no error)"=w341, "Item Tag"=w337, "Execution UI in"=w339) -> ("error out"=w340:errorcluster, "Execution UI out"=w338:refnum<class "Execution UI.lvclass">)  [unwired: 6 in]
              }
              frame "Show Project Item Overlays" {
                n221 = Current VI's Menubar() -> (w342:refnum<k9>)
                n222 = call "Toggle Plugin.vi"("menu reference"=w342, "error in (no error)"=w347, "Item Tag"=w343, "Execution UI in"=w345) -> ("error out"=w346:errorcluster, "Execution UI out"=w344:refnum<class "Execution UI.lvclass">)  [unwired: 6 in]
              }
              frame "Reset" {
                n223 = control-ref of="This VI"() -> (w348:refnum<vi>)
                n224 = call "Initialize Controls and Indicators.vi"("error in (no error)"=w352, "VI in"=w348) -> ("error out"=w353:errorcluster)  [unwired: 9 in]
                n225 = control-ref of="This VI"() -> (w349:refnum<vi>)
                n226 = call "Set Front Panel size.vi"("error in (no error)"=w353, "VI in"=w349) -> ("error out"=w351:errorcluster)  [unwired: 9 in]
              }
              frame "Documentation..." {
                n227 = call-poly <vilib>:"Open URL in Default Browser.vi"("error in (no error)"=w354, "URL"="https://lunit.astemes.com/") -> ("error out"=w355:errorcluster)  [unwired: 4 in, 1 out]
              }
              frame "Report issue..." {
                n228 = call-poly <vilib>:"Open URL in Default Browser.vi"("error in (no error)"=w358, "URL"="https://github.com/astemes/astemes-lunit/issues") -> ("error out"=w359:errorcluster)  [unwired: 4 in, 1 out]
              }
              frame "Post an Idea..." {
                n229 = call-poly <vilib>:"Open URL in Default Browser.vi"("error in (no error)"=w362, "URL"="https://www.vipm.io/post/suggestion/?package_name=astemes_lib_lunit&return_url=/package/astemes_lib_lunit/") -> ("error out"=w363:errorcluster)  [unwired: 4 in, 1 out]
              }
              frame "About" {
                n230 = call "About Dialog.vi"() -> ()  [unwired: 12 in]
              }
              frame "Exit" {
                n231 = call-dynamic "Stop.vi"("error in (no error)"=w370, "Execution UI In"=w371) -> ("error out"=w369:errorcluster, "Execution UI Out"=w368:refnum<class "Execution UI.lvclass">)  [unwired: 8 in]
              }
            }
          }
          event User Event {
            n232 = event-data() -> ()  [unwired: 1 in, 4 out]
          }
          event Panel Close? {
            w379 = TRUE  # Discard?
            n233 = event-data() -> ()  [unwired: 1 in, 4 out]
            n234 = call-dynamic "Stop.vi"("error in (no error)"=w375, "Execution UI In"=w378) -> ("error out"=w376:errorcluster, "Execution UI Out"=w377:refnum<class "Execution UI.lvclass">)  [unwired: 8 in]
            n235 = event-data ("Event Filter Node")("Discard?"=w379) -> ()  [unwired: 1 in, 1 out]
          }
        }
        n236 = call "Handle Errors.vi"("error in (no error)"=w52) -> ("error out"=w51:errorcluster)  [unwired: 10 in]
      }
      n237 = Unbundle By Name(w9) -> ("Result Model"=w21:refnum<class "Result Model.lvclass">, "UI Update Queue"=w20:refnum<queue>)
      n238 = control-ref of="Test Results"() -> (w17:refnum<vi>)
      n239 = property on="Property Node" class="VI"(reference=w19) -> ("Panel"=w18:refnum<vi>)  [unwired: 1 in, 2 out]
      n240 = control-ref of="Progress bar"() -> (w15:refnum<vi>)
      n241 = while {
        tunnel: w14 -> [w37]
        tunnel: w21 -> [w36]
        tunnel: w20 -> [w35]
        tunnel: w18 -> [w33]
        tunnel: w17 -> [w28]
        tunnel: w16 -> [w26]
        tunnel: w15 -> [w25]
        stop <- w34 stop-if-true
        # "UI Update Loop"
        n242 = Dequeue Element(queue=w35, error in (no error)=w37) -> (element=w23:string, error out=w24:errorcluster)  [unwired: 1 in, 2 out]
        n243 = property on="Property Node" class="Pnl"(reference=w33, error in=w24, "DeferPanUpdts"=TRUE ("Defer Panel Updates")) -> (reference out=w27:refnum<vi>, error out=w31:errorcluster)
        n244 = case shown="No Error" w31 {
          selector: w31 -> [w42 w49]
          tunnel: w23 -> [w46 _]
          tunnel: w36 -> [w44 _]
          tunnel: [FALSE TRUE] -> w34
          tunnel: [w42 w49] -> w29
          tunnel: w28 -> [w40 _]
          tunnel: w26 -> [w39 _]
          tunnel: w25 -> [w38 _]
          frame No Error {
            w41 = u32 50  # UI Update Limit
            n245 = call "Get Statistics.vi"("Result Model in"=w44) -> ("Results"=w48:T13)  [unwired: 9 in, 1 out]
            n246 = call "Update Tree.vi"("Filter Fails?"="Filter fails", "Test Tree"=w40, "Result Model"=w44) -> ()  [unwired: 8 in, 1 out]
            n247 = call "Format Result Count Strings.vi"(10:"Results"=w39, 11:"Results"=w48) -> ()  [unwired: 9 in, 1 out]
            n248 = call "Set Progressbar Color.vi"("Progress bar Ref"=w38, "Results"=w48) -> ()  [unwired: 9 in, 1 out]
            n249 = Unbundle By Name(w48) -> ("Progress [%]"=→"Progress bar":dbl)
            n250 = Wait (ms)(milliseconds to wait=w41) -> ()  [unwired: 1 out]
            "Status" <- w46
          }
          frame Error {
          }
        }
        n251 = property on="Property Node" class="Pnl"(reference=w27, error in=w29, "DeferPanUpdts"=FALSE ("Defer Panel Updates")) -> ()  [unwired: 2 out]
      }
      n252 = Merge Errors(w11, w13) -> (w12:errorcluster)
    }
    frame Error {
      n253 = call "Handle Errors.vi"("error in (no error)"=w601) -> ()  [unwired: 10 in, 1 out]
    }
  }
  n254 = Unregister For Events(event registration refnum=w2) -> ()  [unwired: 1 in, 1 out]
  n255 = call <vilib>:"Simple Error Handler.vi"("error in (no error)"=w3) -> ()  [unwired: 4 in, 5 out]
